vi "VeristandStart.vi"(2 "error in (no error)":errorcluster, 3 "Open VeriStand Timeout (s)":i32=120) -> (0 "error out":errorcluster)   [LabVIEW 2015, in "ni-veristand-steps-runtime-lib.lvlib"]
uses:
  ni-veristand-steps-runtime-lib.lvlib
  <vilib>/Utility/sysdir.llb/System Directory Type.ctl
  <vilib>/Utility/error.llb/Error Cluster From Error Code.vi
  <vilib>/ErrorRing/Error Ring.xnode
  <vilib>/NI Veristand/Execution/Workspace/NI_VS Workspace ExecutionAPI.lvlib
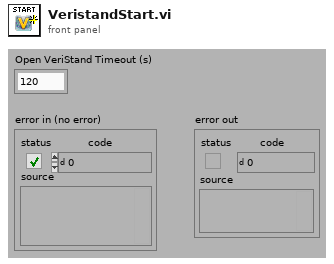
[diagram p1: front panel]
types:
  T1 = typedef "System Directory Type.ctl" = i32
  T2 = typedef "NI_VS Workspace ExecutionAPI.lvlib/WorkspaceAPI.ctl" = refnum<k24>
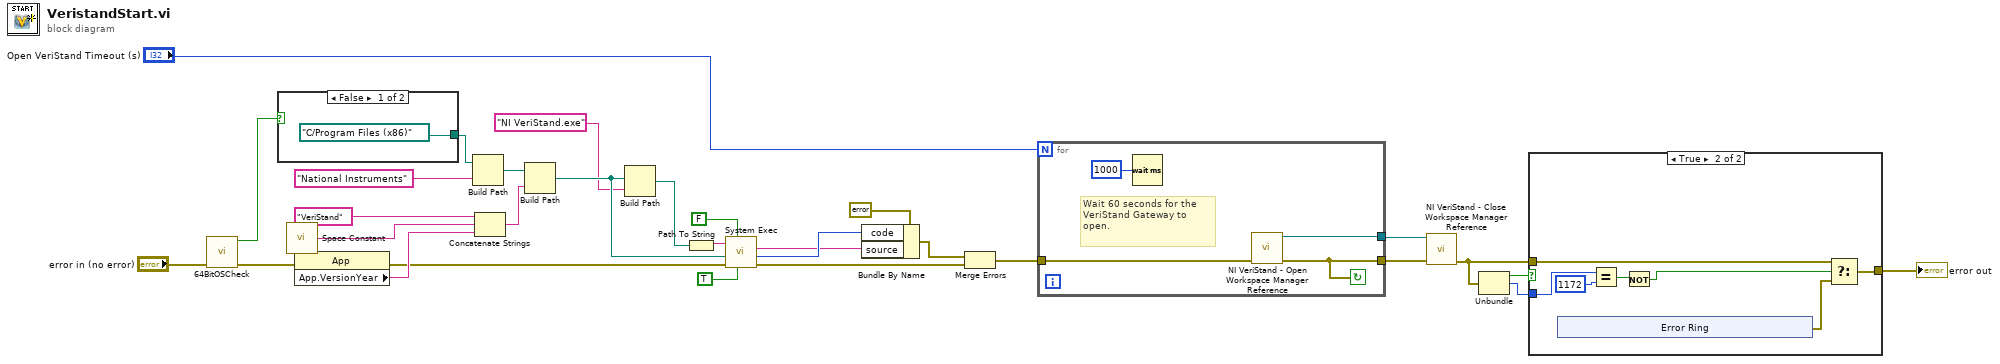
[diagram p0: block diagram]
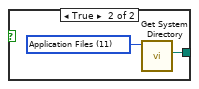
[diagram p3: hidden frame]
diagram:
  n1 = call "64BitOSCheck.vi"("error in (no error)"="error in (no error)") -> ("error out"=w9:errorcluster, "Is64Bit?"=w11:bool)  [unwired: 9 in]
  n2 = case shown="False" w11 {
    tunnel: [path "C:/Program Files (x86)" ("system directory") w32] -> w29
    frame False {
    }
    frame True {
      w33 = T1 11 items=["User Home"=0, "User Desktop"=1, "User Documents"=2, "User Application Data"=3, "User Preferences"=4, "User Temporary"=5, "Public Documents"=6, "Public Application Data"=7, "Public Preferences"=8, "Public Cache"=13, "System Core Libraries"=9, "System Installed Libraries"=10, "Application Files"=11, "Boot Volume Root"=12] ("system directory type")
      n3 = call <vilib>:"Get System Directory.vi"("system directory type"=w33) -> ("system directory"=w32:path)  [unwired: 10 in]
    }
  }
  n4 = call <vilib>:"Space Constant.vi"() -> ("String"=w22:string)
  n5 = property class="App"(error in=w9) -> (error out=w12:errorcluster, "App.VersionYear"=w23:string)  [unwired: 1 in, 1 out]
  n6 = Build Path(base path=w29, name or relative path="National Instruments") -> (appended path=w27:path)
  n7 = Concatenate Strings("VeriStand" ("name or relative path"), w22, w23) -> (w21:string)
  n8 = Build Path(base path=w27, name or relative path=w21) -> (appended path=w20:path)
  n9 = Build Path(base path=w20, name or relative path="NI VeriStand.exe") -> (appended path=w26:path)
  n10 = Path To String(path=w26) -> (string=w25:string)
  n11 = call <vilib>:"System Exec.vi"("run minimized? (F)"=TRUE, "wait until completion? (T)"=FALSE, "error in (no error)"=w12, "working directory"=w20, "command line"=w25) -> ("error out"=w15:errorcluster, "return code"=w17:i32, "standard error"=w14:string)  [unwired: 3 in, 1 out]
  n12 = Bundle By Name(cluster=errorcluster {"status"=FALSE, "code"=0, "source"=""} ("error in (no error)"), "code"=w17, "source"=w14) -> (w16:errorcluster)
  n13 = Merge Errors(w16, w15) -> (w7:errorcluster)
  n14 = for {
    N: "Open VeriStand Timeout (s)" -> [_]
    tunnel: [w35] -> w6
    tunnel: w7 -> [w34]
    tunnel: [w36] -> w8
    stop <- w36 continue-if-true
    # "Wait 60 seconds for the VeriStand Gateway to open."
    n15 = Wait (ms)(milliseconds to wait=u32 1000) -> ()  [unwired: 1 out]
    n16 = call <vilib>:"NI VeriStand - Open Workspace Manager Reference.vi"("error in (no error)"=w34) -> ("error out"=w36:errorcluster, "WorkspaceManager"=w35:T2)  [unwired: 9 in]
  }
  n17 = call <vilib>:"NI VeriStand - Close Workspace Manager Reference.vi"("error in (no error)"=w8, "WorkspaceManager"=w6) -> ("error out"=w4:errorcluster)  [unwired: 9 in]
  n18 = Unbundle(w4) -> ("status"=w5:bool, "code"=w3:i32)  [unwired: 1 out]
  n19 = case shown="True" w5 {
    tunnel: w3 -> [_ w45]
    tunnel: w4 -> [w38 w42]
    tunnel: [w38 w43] -> w2
    frame False {
    }
    frame True {
      n20 = xnode "Error Ring"() -> ("error out"=w39:errorcluster)
      n21 = Equal?(x=w45, y=1172) -> (x = y?=w41:bool)
      n22 = Not(x=w41) -> (.not. x?=w40:bool)
      n23 = Select(t=w42, s=w40, f=w39) -> (s? t:f=w43:errorcluster)
    }
  }
  "error out" <- w2
